vi "Initialization VI.vi"(8 "error in (no error)":errorcluster, 10 "Custom XML":string, 11 "Device Item Ref in":T1 format="%.0x") -> (0 "error out":errorcluster, 3 "Device Item Ref out":T1 format="%.0x")   [LabVIEW 2019, in "RefMem DMA System Explorer.lvlib"]
uses:
  RefMem DMA System Explorer.lvlib
  <vilib>/NI VeriStand/Custom Device API/Custom Device Item Ref.ctl
  <vilib>/NI VeriStand/Custom Device API/Custom Device Channel.ctl
  <vilib>/NI VeriStand/Custom Device API/Custom Device Channel Type.ctl
  <vilib>/NI VeriStand/Custom Device API/Custom Device Loop Type.ctl
  Shared/Constants.vi
  <vilib>/NI VeriStand/Custom Device API/Custom Device API.lvlib
  Shared/RefMem DMA Shared.lvlib
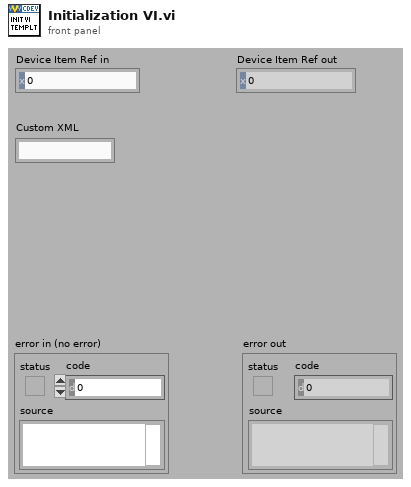
[diagram p1: front panel]
types:
  T1 = typedef "Custom Device API.lvlib/Custom Device Item Ref.ctl" = u64
  T2 = typedef "Custom Device API.lvlib/Custom Device Loop Type.ctl" = enum32{"While Loop", "Timed Loop"}
  T3 = typedef "Custom Device API.lvlib/Custom Device Channel.ctl" = cluster{"Type":T4, "Units":string, "Default Value":dbl, "Faultable":bool, "Scalable":bool}
  T4 = typedef "Custom Device API.lvlib/Custom Device Channel Type.ctl" = enum16{"Input", "Output"}
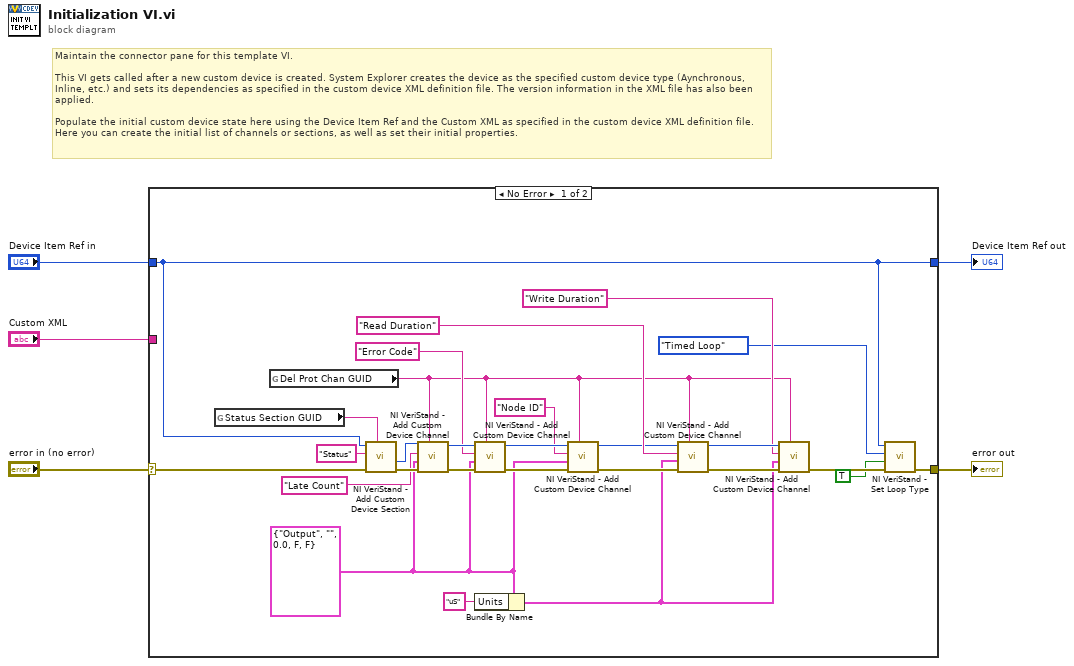
[diagram p0: block diagram]
diagram:
  # "Maintain the connector pane for this template VI.\n\nThis VI gets called after a new custom device is created. System Explorer creates the device as the specified custom device type (Aynchronous, Inline, etc.) and sets its dependencies as specified in the custom device XML definition file. The version information in the XML file has also been applied.\n\nPopulate the initial custom device state here using the Device Item Ref and the Custom XML as specified in the custom device XML definition file. Here you can create the initial list of channels or sections, as well as set their initial properties."
  n1 = case shown="No Error" "error in (no error)" {
    selector: "error in (no error)" -> [w29 w34]
    tunnel: [w9 w34] -> w5
    tunnel: [w6 w33] -> w3
    tunnel: "Device Item Ref in" -> [w6 w33]
    tunnel: "Custom XML" -> [_ _]
    frame No Error {
      w16 = T3 {"Type"=enum."Output", "Units"="", "Default Value"=0.0, "Faultable"=FALSE, "Scalable"=FALSE} ("Channel")
      n2 = global read "Constants.vi" "Status Section GUID"() -> (w27:string)
      n3 = global read "Constants.vi" "Del Prot Chan GUID"() -> (w12:string)
      n4 = call <vilib>:"NI VeriStand - Add Custom Device Section.vi"("GUID (Default Section)"=w27, "error in (no error)"=w29, "Section Name"="Status", "Parent Ref in"=w6) -> ("error out"=w32:errorcluster, "Section Ptr"=w30:T1)  [unwired: 4 in, 2 out]
      n5 = call <vilib>:"NI VeriStand - Add Custom Device Channel.vi"("GUID (Default Channel)"=w12, "error in (no error)"=w32, "Channel"=w16, "Channel Name"="Late Count", "Parent Ref in"=w30) -> ("error out"=w22:errorcluster, "Parent Ref out"=w31:T1)  [unwired: 3 in, 2 out]
      n6 = call <vilib>:"NI VeriStand - Add Custom Device Channel.vi"("GUID (Default Channel)"=w12, "error in (no error)"=w22, "Channel"=w16, "Channel Name"="Error Code", "Parent Ref in"=w31) -> ("error out"=w21:errorcluster, "Parent Ref out"=w19:T1)  [unwired: 3 in, 2 out]
      n7 = Bundle By Name(cluster=w16, "Units"="uS") -> (w11:T3)
      n8 = call <vilib>:"NI VeriStand - Add Custom Device Channel.vi"("GUID (Default Channel)"=w12, "error in (no error)"=w21, "Channel"=w16, "Channel Name"="Node ID", "Parent Ref in"=w19) -> ("error out"=w20:errorcluster, "Parent Ref out"=w18:T1)  [unwired: 3 in, 2 out]
      n9 = call <vilib>:"NI VeriStand - Add Custom Device Channel.vi"("GUID (Default Channel)"=w12, "error in (no error)"=w20, "Channel"=w11, "Channel Name"="Read Duration", "Parent Ref in"=w18) -> ("error out"=w15:errorcluster, "Parent Ref out"=w14:T1)  [unwired: 3 in, 2 out]
      n10 = call <vilib>:"NI VeriStand - Add Custom Device Channel.vi"("GUID (Default Channel)"=w12, "error in (no error)"=w15, "Channel"=w11, "Channel Name"="Write Duration", "Parent Ref in"=w14) -> ("error out"=w10:errorcluster)  [unwired: 3 in, 3 out]
      n11 = call <vilib>:"NI VeriStand - Set Loop Type.vi"("error in (no error)"=w10, "Use Device Clock (Timed Loops only)"=TRUE, "Loop type"=Custom_Device_Loop_Type."Timed Loop", "Device Ref in"=w6) -> ("error out"=w9:errorcluster)  [unwired: 6 in, 1 out]
    }
    frame Error {
    }
  }
  "error out" <- w5
  "Device Item Ref out" <- w3
